vi "Radio Buttons - Entire Dataset for desired quantity.vi"() -> ()   [LabVIEW 2020]
panel:
  out "XY Graph":cluster{dbl[], dbl[]}(graph)
  out "output array":dbl[][](array[numeric])
  out "Intensity Graph":dbl[][](graph)
  in  "Radio Buttons":T1(radio)=enum."Peak Positive"
  in  "Rows":dbl
  in  "Columns":dbl
  in  "Path":path=path "C:/Users/gaeta/Desktop/Unif Leerstof/Individual Project/Osc. Data/wetransfer-86c2d3/2DZXaxisscan 0.28MHz 30x30mm 20mvpp 1020L centre 390mm from td plane.mat"
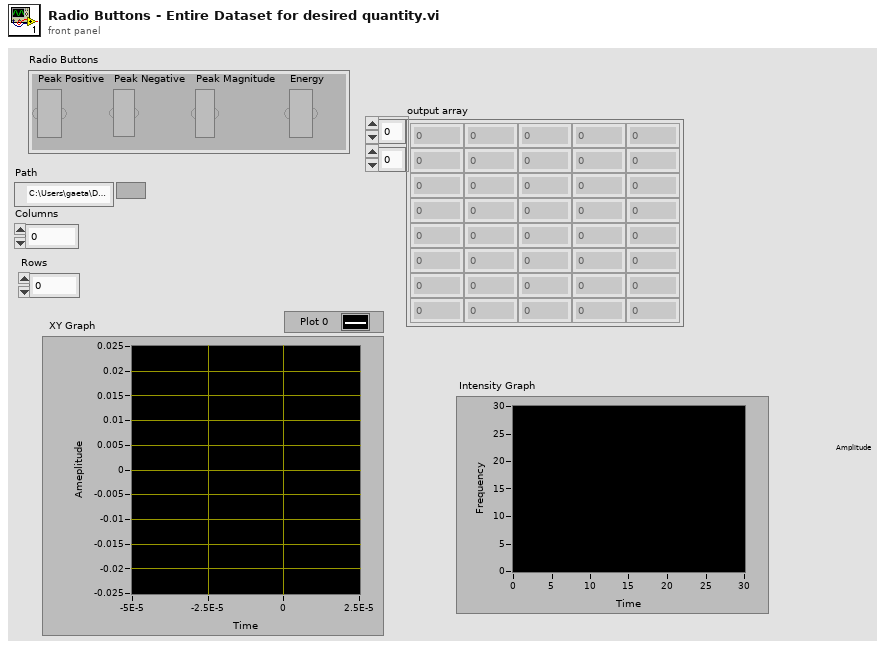
[diagram p1: front panel]
types:
  T1 = enum32{"No Selection", "Peak Positive", "Peak Negative", "Peak Magnitude", "Energy"}
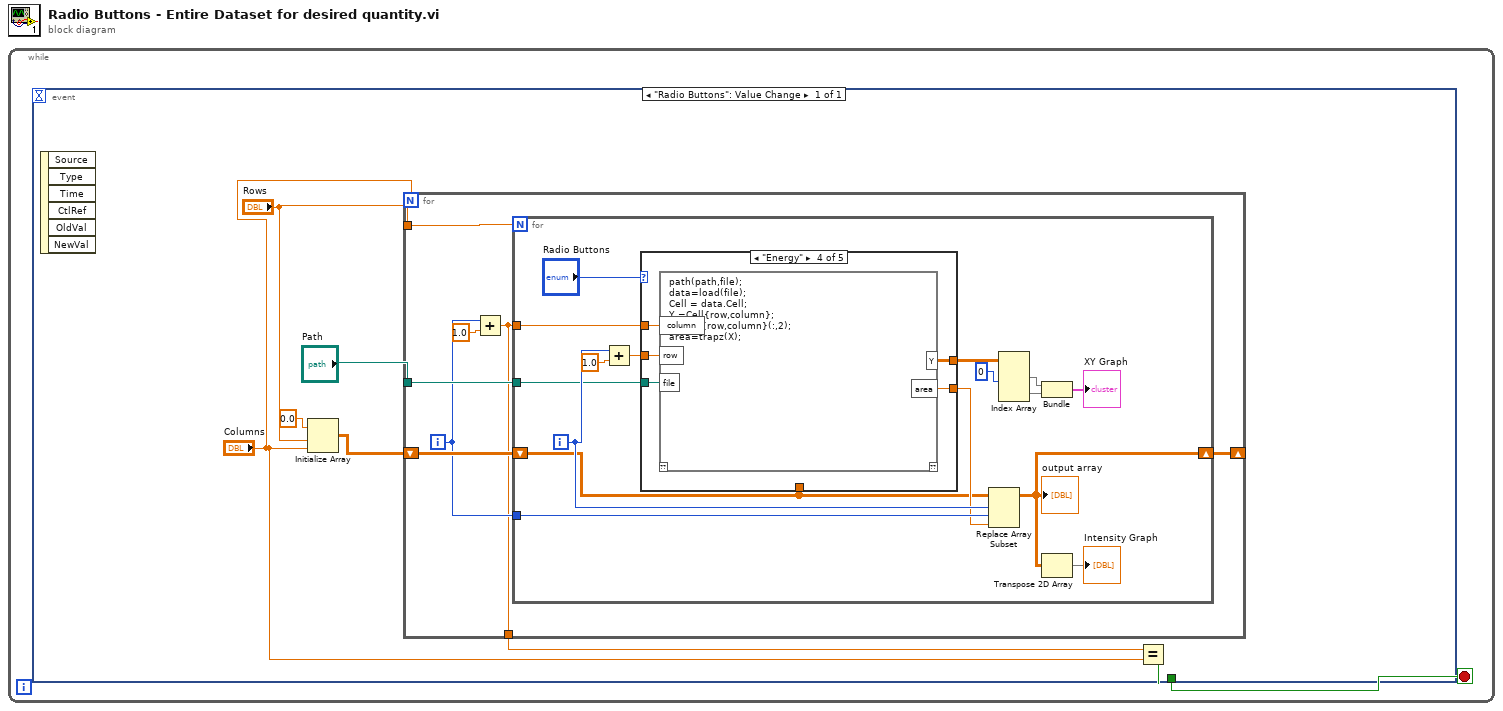
[diagram p0: block diagram]
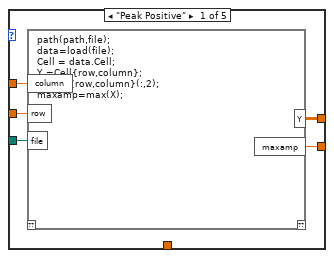
[diagram p2: hidden frame]
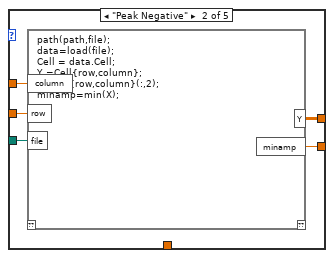
[diagram p3: hidden frame]
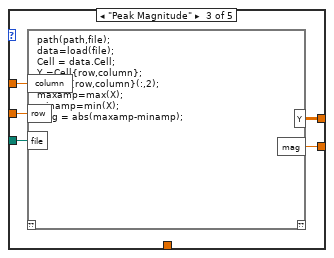
[diagram p4: hidden frame]
diagram:
  n1 = while {
    stop <- w1 stop-if-true
    n2 = event shown="[0] \"Radio Buttons\": Value Change" {
      selector: _ -> [_]
      dyn-events: _ -> [_]
      timeout: _ -> [_]
      tunnel: [w2] -> w1
      event "Radio Buttons": Value Change {
        n3 = event-data() -> ()  [unwired: 1 in, 6 out]
        n4 = Initialize Array(0.0 ("element"), "Rows", "Columns") -> (w5:dbl[][])
        n5 = for {
          N: "Columns" -> [_]
          tunnel: "Path" -> [w15]
          tunnel: "Rows" -> [w13]
          shift-right: [w11] -> _
          shift-left: w5 -> [w12]
          tunnel: [w9] -> w3
          i -> [w10]
          n6 = Add(x=w10, y=1.0) -> (x+y=w9:dbl)
          n7 = for {
            N: w13 -> [_]
            tunnel: w15 -> [w21]
            tunnel: w9 -> [w23]
            shift-right: [w26] -> w11
            shift-left: w12 -> [w17]
            tunnel: w10 -> [w24]
            i -> [w27]
            n8 = Add(x=w27, y=1.0) -> (x+y=w22:dbl)
            n9 = case shown="\"Energy\"" "Radio Buttons" {
              tunnel: w23 -> [w32 w37 w42 w47 _]
              tunnel: w22 -> [w36 w41 w44 w49 _]
              tunnel: w21 -> [w35 w40 w43 w48 _]
              tunnel: [w33 w39 w45 w50 _] -> w20
              tunnel: [w34 w38 w46 w51 _] -> w19
              tunnel: w17 -> [_ _ _ _ _]
              frame "Peak Positive" {
                n10 = script code="path(path,file);\ndata=load(file);\nCell = data.Cell;\nY =Cell{row,column};\nX=Cell{row,column}(:,2);\nmaxamp=max(X);"("row"=w36, "file"=w35, "column"=w32) -> ("Y"=w34:dbl[][], "maxamp"=w33:dbl)  [unwired: 1 in, 1 out]
              }
              frame "Peak Negative" {
                n11 = script code="path(path,file);\ndata=load(file);\nCell = data.Cell;\nY =Cell{row,column};\nX=Cell{row,column}(:,2);\nminamp=min(X);"("row"=w41, "file"=w40, "column"=w37) -> ("Y"=w38:dbl[][], "minamp"=w39:dbl)  [unwired: 1 in, 1 out]
              }
              frame "Peak Magnitude" {
                n12 = script code="path(path,file);\ndata=load(file);\nCell = data.Cell;\nY =Cell{row,column};\nX=Cell{row,column}(:,2);\nmaxamp=max(X);\nminamp=min(X);\nmag = abs(maxamp-minamp);"("row"=w44, "file"=w43, "column"=w42) -> ("Y"=w46:dbl[][], "mag"=w45:dbl)  [unwired: 1 in, 1 out]
              }
              frame "Energy" {
                n13 = script code="path(path,file);\ndata=load(file);\nCell = data.Cell;\nY =Cell{row,column};\nX=Cell{row,column}(:,2);\narea=trapz(X);"("row"=w49, "file"=w48, "column"=w47) -> ("Y"=w51:dbl[][], "area"=w50:dbl)  [unwired: 1 in, 1 out]
              }
              frame "No Selection" {
              }
            }
            n14 = Replace Array Subset(array=w17, new element=w20, index (row)=w27, index (col)=w24) -> (w26:dbl[][])
            "output array" <- w26
            n15 = Index Array(array=w19, index (col) #1=0 ("disabled index (col)")) -> (element #1=w29:dbl[], element #2=w30:dbl[])  [unwired: 3 in]
            n16 = Bundle(w29, w30) -> (→"XY Graph":cluster{dbl[], dbl[]})  [unwired: 1 in]
            n17 = Transpose 2D Array(2D array=w26) -> (transposed array=→"Intensity Graph":dbl[][])
          }
        }
        n18 = Equal?(x=w3, y="Columns") -> (x = y?=w2:bool)
      }
    }
  }
